vi "Get Name.vi"(11 "Transfer in":refnum<class "Transfer.lvclass">) -> (2 "name":string, 3 "Transfer out":refnum<class "Transfer.lvclass">)   [LabVIEW 2019, in "DSF Core.lvlib" / "Transfer.lvclass"]
uses:
  Transfer.lvclass
  Transfer.lvclass/Transfer.ctl
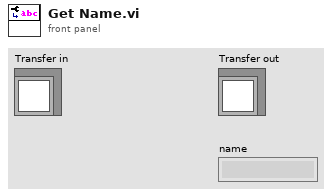
[diagram p1: front panel]
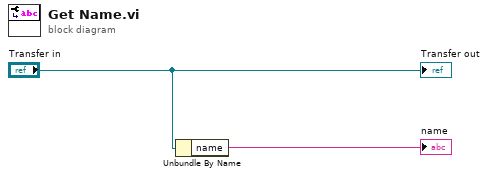
[diagram p0: block diagram]
diagram:
  n1 = Unbundle By Name("Transfer in") -> ("name"=→"name":string)
  "Transfer out" <- "Transfer in"
